vi "Кластер числовых параметров мишени в строку (SubVI).vi"(1 "Кластер числовых параметров мишени":T1) -> (0 "Строка числовых парам. мишени + переход на новую сторку":string)   [LabVIEW 2015]
doc: "Преобразует числовые параметры мишени в строку для дальнейшего сохранения в файл"
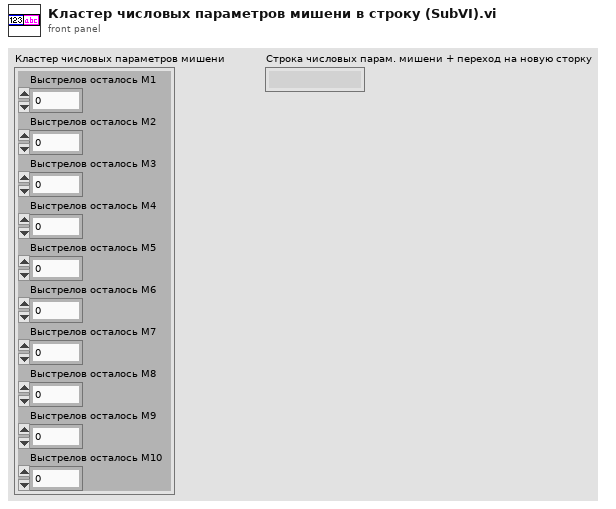
[diagram p1: front panel]
types:
  T1 = cluster{"Выстрелов осталось M1 ":u16, "Выстрелов осталось M2":u16, "Выстрелов осталось M3":u16, "Выстрелов осталось M4":u16, "Выстрелов осталось M5":u16, "Выстрелов осталось M6":u16, "Выстрелов осталось M7":u16, "Выстрелов осталось M8":u16, "Выстрелов осталось M9":u16, "Выстрелов осталось M10":u16}
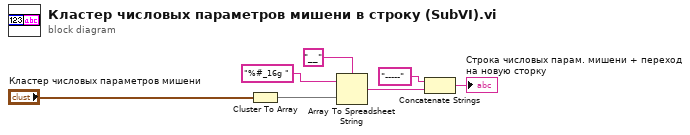
[diagram p0: block diagram]
diagram:
  n1 = Cluster To Array(cluster="Кластер числовых параметров мишени") -> (array=w6:u16[])
  n2 = Array To Spreadsheet String(delimiter (Tab)="__", array=w6, 3:"%#_16g " ("format string")) -> (spreadsheet string=w3:string)
  n3 = Concatenate Strings("-----" ("regular expression"), w3) -> (→"Строка числовых парам. мишени + переход на новую сторку":string)
